vi "主程序-复材超声C扫缺陷分析评定软件.vi"() -> ()   [LabVIEW 2018]
doc: "使用该模板构建用户界面事件处理设计模式。将模板应用于对话框及其它用户界面。用户也可创建并执行VI可按照与用户界面事件相同方式处理的用户定义事件。"
uses:
  <vilib>/Utility/NIReport.llb/Report Type.ctl
  <vilib>/addons/_office/_exclsub.llb/font.ctl
  <vilib>/Utility/NIReport.llb/HTML Report Image Alignment.ctl
  <vilib>/Utility/NIReport.llb/Append Report Text (str wrap).vi
  <vilib>/Utility/NIReport.llb/Append Image to Report (path wrap).vi
  <vilib>/addons/_office/word.llb/Word Easy Table (str).vi
  <vilib>/Utility/NIReport.llb/NI_report.lvclass
  <vilib>/Utility/NIReport.llb/Word/NI_Word.lvclass
  <vilib>/addons/_office/NI_ReportGenerationToolkit.lvlib
  <vilib>/Utility/NIReport.llb/NI_ReportGenerationCore.lvlib
  <vilib>/vision/NI_Vision_Development_Module.lvlib
panel:
  out "框号字体大小-":i16
  out "是否需要预处理":u16
  out "弥散类缺陷灰度阈值":dbl caption="值"
  out "计入分层缺陷的面积阈值":i32
  out "报告模式":string
  in  "删除标注":bool caption="定量分析"
  out "分层类缺陷灰度阈值":dbl caption="值"
  out "反射图原始路径":path
  out "穿透图原始路径":path
  out "ROImask":T1(plugin-control)
  out "模式选择":u16(ring) items=["只读穿透图", "穿透图和反射图结合"]
  out "添加的路径":path
  out "连接的字符串 2":string
  out "临界面积百分比值":dbl
  out "临界Z值":i32
  out "标注后的图片路径":path
  out "全部检测结果合并":string[][](table)
  out "全部检测结果":string[][](table)
  out "部位信息":string[](array[string])=["", "34.500000", "32.500000", "1121", "34", "54.955926", "分层类", "不合格", ""]
  out "连接的字符串":string
  in  "完成标注":bool caption="定量分析"
  out "框数":dbl
  out "自定义字体":T2={"Desired Font (Application)"=enum."Application Font", "[User-specified Font]"={"Font Name"="", "Size"=12, "Strikeout?"=FALSE, "Italic?"=FALSE, "Underline?"=FALSE, "Outline?"=FALSE, "Shadow?"=FALSE, "Bold?"=FALSE, "Rotation Angle"=0.0}, "Horizontal Alignment"=0, "Vertical Alignment"=0} {"Horizontal Alignment" items=["Left", "Center", "Right"]; "Vertical Alignment" items=["Bottom", "Top", "Baseline"]}
  out "框组":T3(array[cluster])
  out "质量等级":string
  in  "stop":bool caption="停止"
  in  "导入图像":bool caption="导入图片"
  in  "开始标注":bool caption="定量分析"
  in  "查看评定结果":bool caption="辅助定性分析"
  in  "生成报告":bool caption="生成原始记录"
  in  "控件":enum32{"穿透图", "反射图"}(tab)
  out "穿透图":T1(plugin-control)
  out "反射图":T1(plugin-control)
  out "产品规格":cluster{"产品长度（周长）（mm）":dbl, "产品宽度（母线长）（mm）":dbl}
  out "图像分辨率":T4
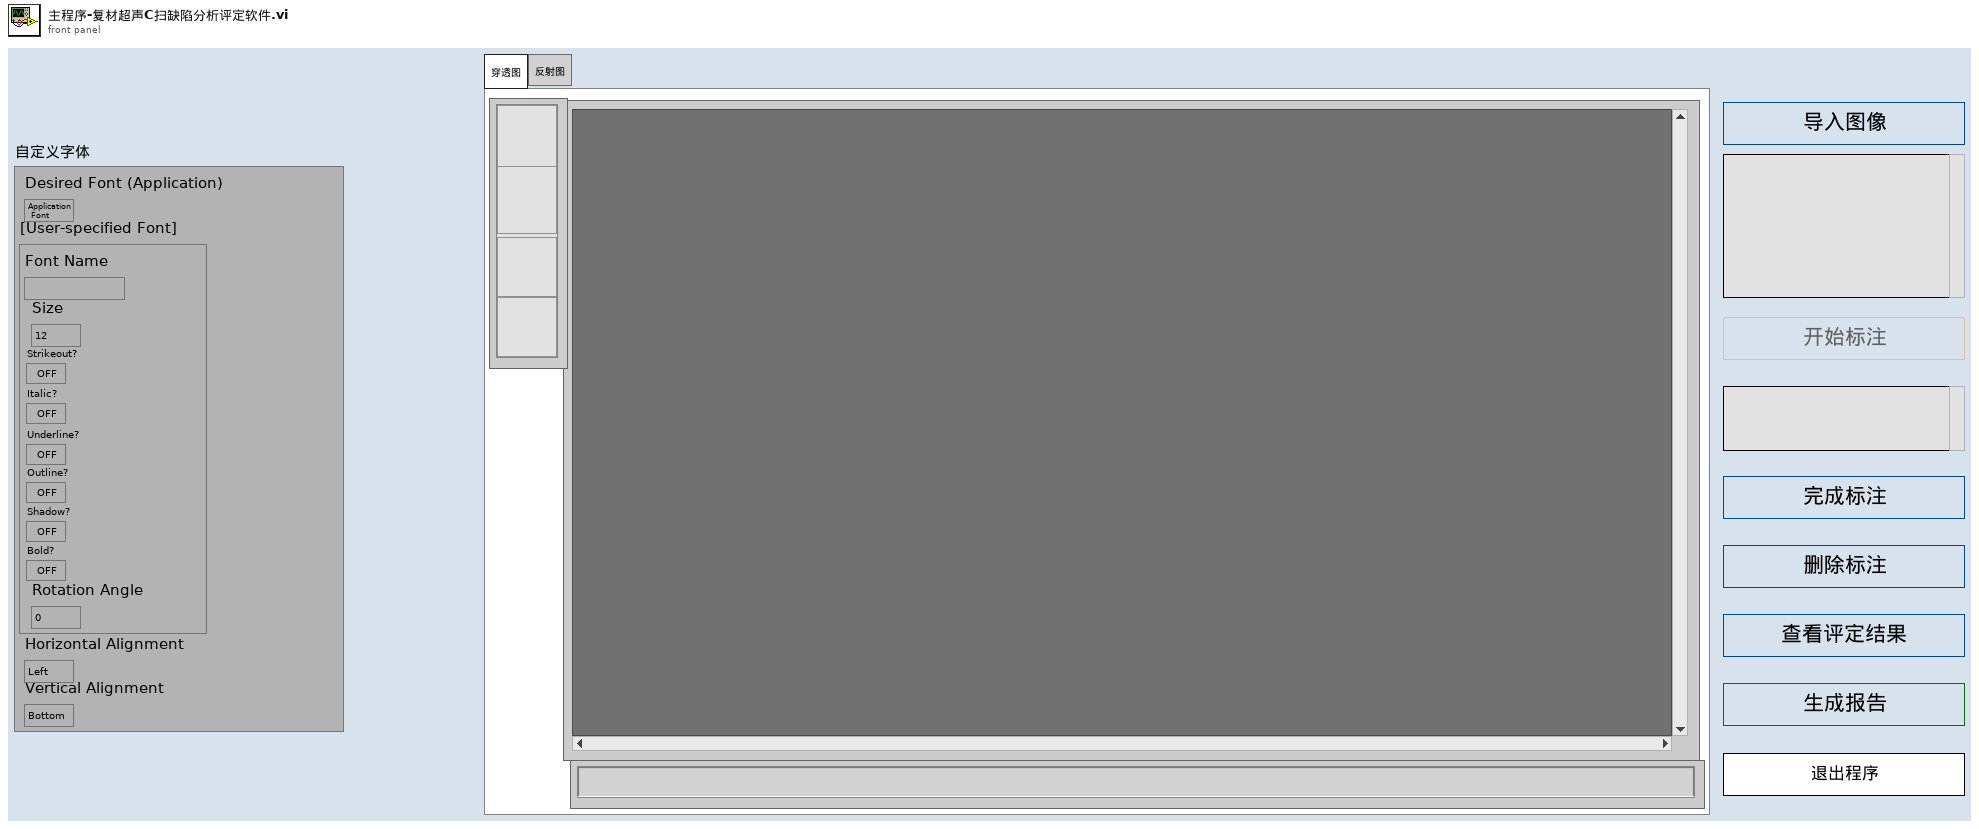
[diagram p1: front panel]
types:
  T1 = typedef "IMAQ Image.ctl" = refnum<image>
  T2 = cluster{"Desired Font (Application)":enum16{"User-specified Font", "Application Font", "System Font", "Dialog Font"}, "[User-specified Font]":cluster{"Font Name":string, "Size":i16, "Strikeout?":bool, "Italic?":bool, "Underline?":bool, "Outline?":bool, "Shadow?":bool, "Bold?":bool, "Rotation Angle":dbl}, "Horizontal Alignment":i16, "Vertical Alignment":i16}
  T3 = cluster{"Global Rectangle":i32[], "Contours":cluster{"Contour Type":u32, "ROI Type":u32, "Points":i32[]}[]}[]
  T4 = cluster{"图像X向分辨率（mm/像素）":dbl, "图像Y向分辨率（mm/像素）":dbl}
  T5 = enum8{"Enabled", "Disabled", "Disabled and Grayed Out"}
  T6 = cluster{"Global Rectangle":i32[], "Contours":cluster{"Contour Type":u32, "ROI Type":u32, "Points":i32[]}[]}
  T7 = cluster{"Zoom Tool":bool, "Selection Tool":bool, "Pan Tool":bool, "Point Tool":bool, "Line Tool":bool, "Rectangle Tool":bool, "Rotated Rectangle Tool":bool, "Polyline Tool":bool, "Polygon Tool":bool, "Freehand Tool":bool, "Closed Freehand Tool":bool, "Ellipse Tool":bool, "Annulus Tool":bool}
  T8 = enum16{"maximized", "minimized", "normal", "no change"}
  T9 = typedef "NI_ReportGenerationCore.lvlib/Report Type.ctl" = enum16{"HTML", "Word", "Excel"}
  T10 = typedef "NI_ReportGenerationCore.lvlib/HTML Report Image Alignment.ctl" = enum16{"(default)", "LEFT", "RIGHT", "TOP", "TEXTTOP", "MIDDLE", "ABSMIDDLE", "BASELINE", "BOTTOM", "ABSBOTTOM"}
  T11 = cluster{"position (Excel)":cluster{"row":i32, "column":i32}, "name (Excel)":string, "bookmark (Word)":string}
  T12 = cluster{"position (excel)":cluster{"row":i32, "column":i32}, "name (excel)":string, "bookmark (word)":string}
  T13 = typedef "NI_ReportGenerationToolkit.lvlib/font.ctl" = cluster{"font name":string, "font size":dbl, "bold":u16, "italic":u16, "underline":u16, "strike through":u16, "font color":u32}
  T14 = typedef "Image Type" = u32
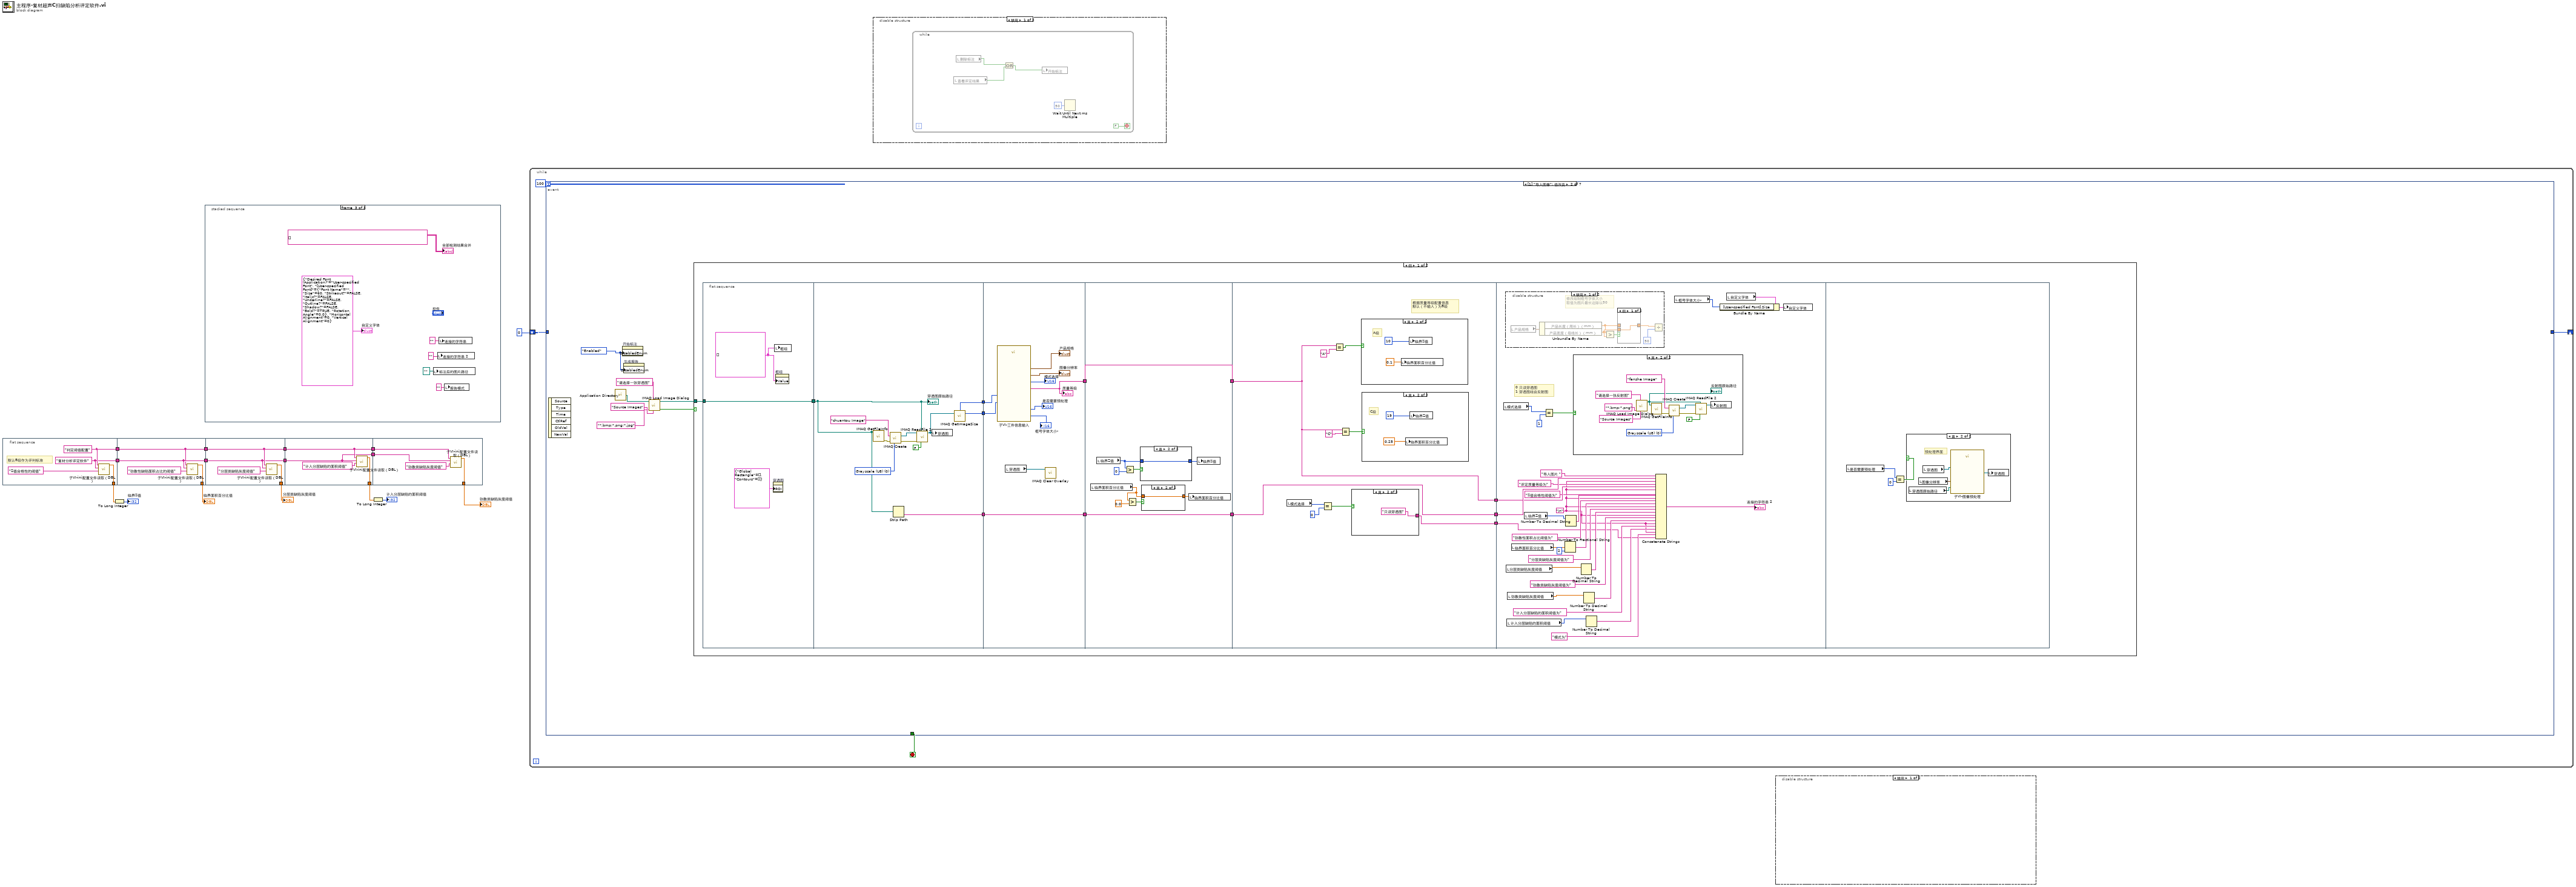
[diagram p0: block diagram]
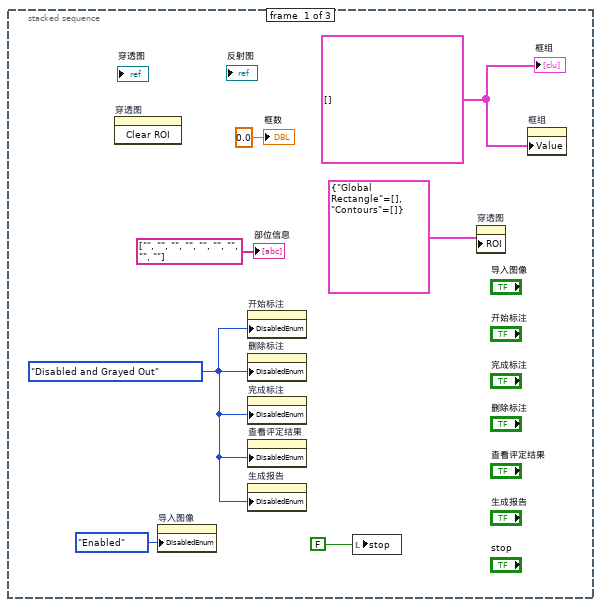
[diagram p3: hidden frame]
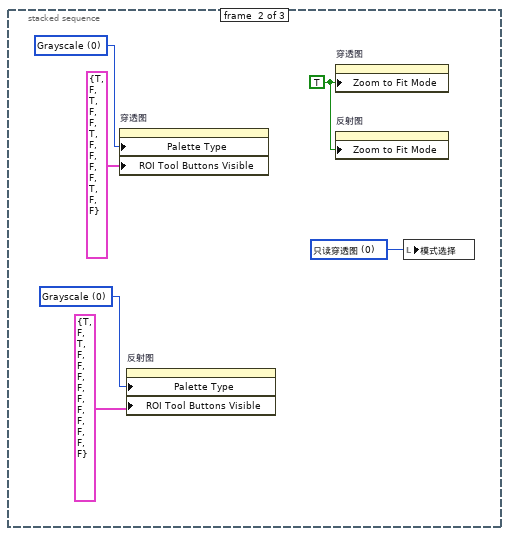
[diagram p4: hidden frame]
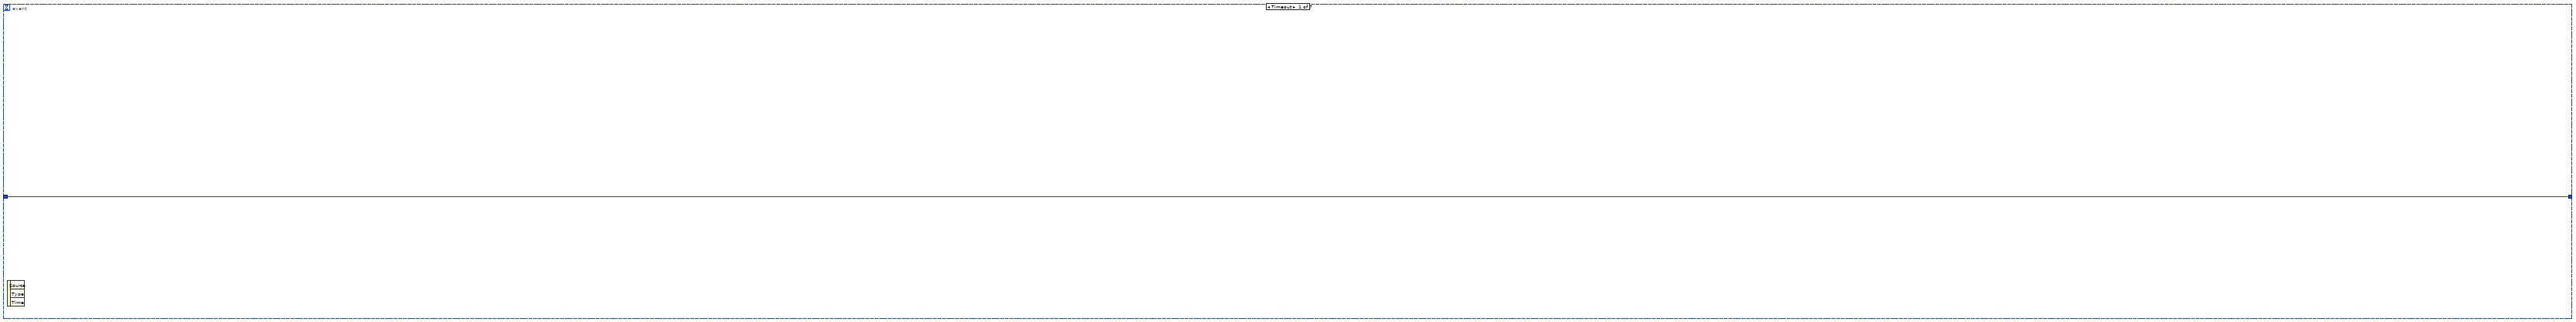
[diagram p6: hidden frame]
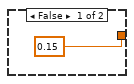
[diagram p7: hidden frame]
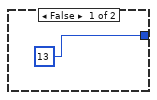
[diagram p8: hidden frame]
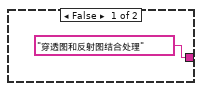
[diagram p9: hidden frame]
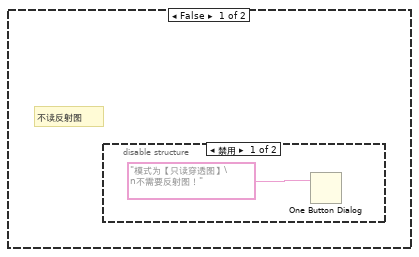
[diagram p14: hidden frame]
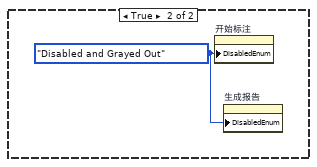
[diagram p17: hidden frame]
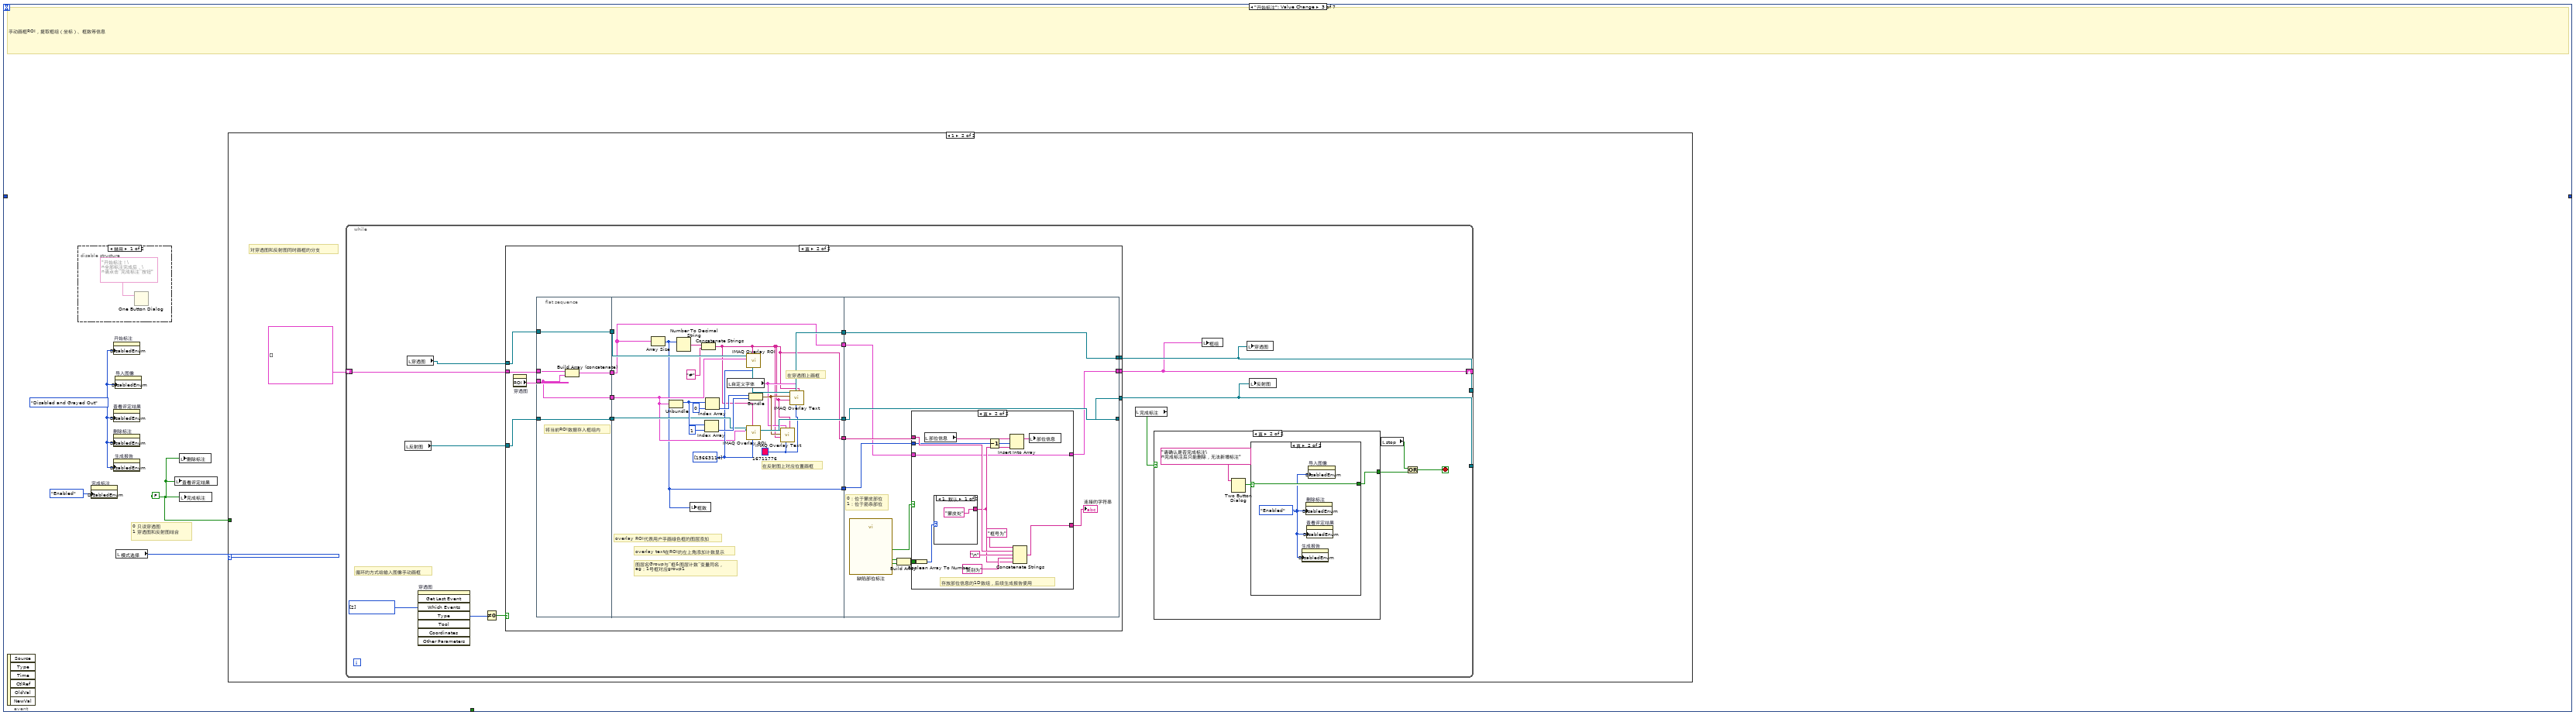
[diagram p18: hidden frame]
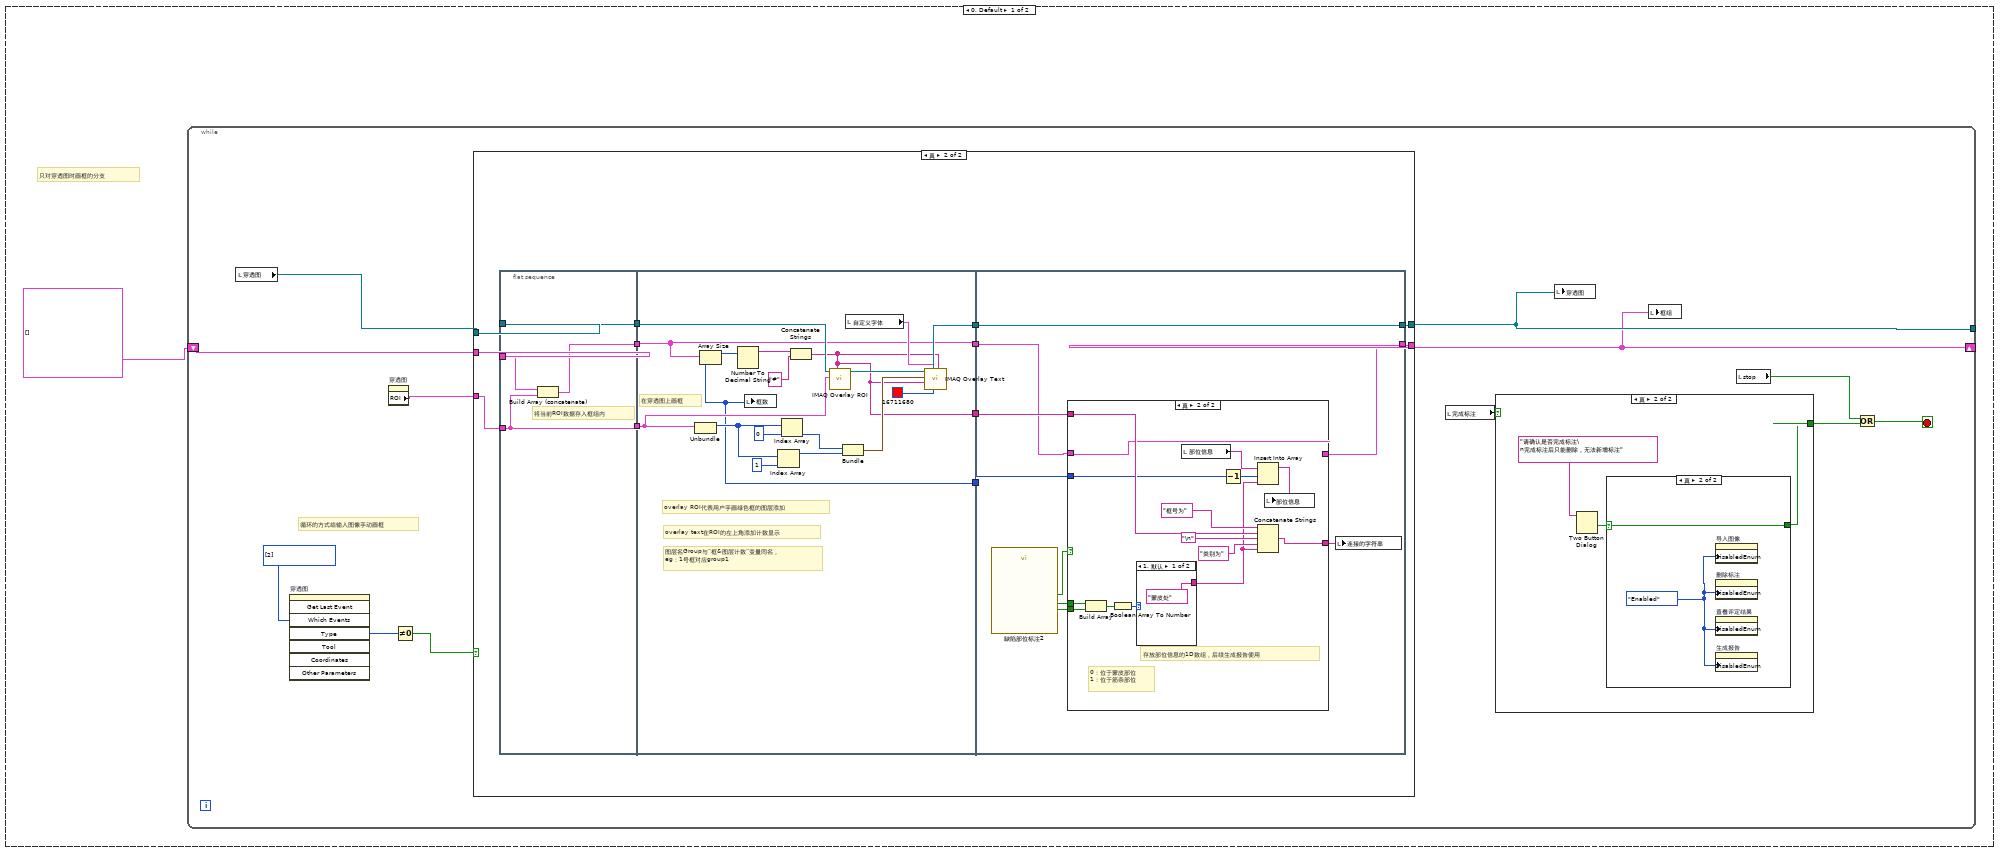
[diagram p20: hidden frame]
diagram:
  n1 = flat-sequence {
    tunnel: [w19] -> w15
    tunnel: [w18] -> w14
    tunnel: [w17] -> w9
    tunnel: w15 -> [w22]
    tunnel: w14 -> [w23]
    tunnel: [w23] -> w13
    tunnel: [w22] -> w12
    tunnel: [w21] -> w10
    tunnel: w13 -> [w25]
    tunnel: w12 -> [w26]
    tunnel: [w27] -> w11
    tunnel: [w26] -> w7
    tunnel: [w25] -> w6
    tunnel: w7 -> [w30]
    tunnel: w6 -> [w29]
    tunnel: [w31] -> w4
    tunnel: [w30] -> w3
    tunnel: [w29] -> w2
    tunnel: w3 -> [w35]
    tunnel: w2 -> [w34]
    tunnel: [w33] -> w1
    frame #0 {
      w18 = "复材分析评定软件" ("section")
      w19 = "判定阈值配置" ("文件名称")
      # "默认B级作为评判标准"
      n2 = call "子VI-ini配置文件读取（DBL）.vi"("key"="Z值合格性的阈值", "section"=w18, "文件名称"=w19) -> ("value"=w17:dbl)  [unwired: 8 in]
    }
    frame #1 {
      n3 = call "子VI-ini配置文件读取（DBL）.vi"("key"="弥散性缺陷面积占比的阈值", "section"=w23, "文件名称"=w22) -> ("value"=w21:dbl)  [unwired: 8 in]
    }
    frame #2 {
      n4 = call "子VI-ini配置文件读取（DBL）.vi"("key"="分层类缺陷灰度阈值", "section"=w25, "文件名称"=w26) -> ("value"=w27:dbl)  [unwired: 8 in]
    }
    frame #3 {
      n5 = call "子VI-ini配置文件读取（DBL）.vi"("key"="计入分层缺陷的面积阈值", "section"=w29, "文件名称"=w30) -> ("value"=w31:dbl)  [unwired: 8 in]
    }
    frame #4 {
      n6 = call "子VI-ini配置文件读取（DBL）.vi"("key"="弥散类缺陷灰度阈值", "section"=w34, "文件名称"=w35) -> ("value"=w33:dbl)  [unwired: 8 in]
    }
  }
  n7 = To Long Integer(number=w9) -> (32bit integer=→"临界Z值":i32)
  n8 = stacked-sequence {
    frame #0 {
      w41 = T3 [] ("框组")
      w38 = T5."Disabled and Grayed Out" ("禁用")
      n9 = invoke on="穿透图" class="ImageControl" method="Clear ROI"() -> ()  [unwired: 3 in, 3 out]
      n10 = property on="导入图像" class="Bool"("DisabledEnum"=T5."Enabled" ("禁用")) -> ()  [unwired: 2 in, 2 out]
      n11 = property on="开始标注" class="Bool"("DisabledEnum"=w38) -> ()  [unwired: 2 in, 2 out]
      n12 = property on="删除标注" class="Bool (严格)"("DisabledEnum"=w38) -> ()  [unwired: 2 in, 2 out]
      n13 = property on="完成标注" class="Bool (严格)"("DisabledEnum"=w38) -> ()  [unwired: 2 in, 2 out]
      n14 = property on="查看评定结果" class="Bool (严格)"("DisabledEnum"=w38) -> ()  [unwired: 2 in, 2 out]
      n15 = property on="生成报告" class="Bool"("DisabledEnum"=w38) -> ()  [unwired: 2 in, 2 out]
      n16 = local write "stop"(FALSE ("stop")) -> ()
      n17 = property on="穿透图" class="ImageControl"("ROI"=T6 {"Global Rectangle"=[], "Contours"=[]}) -> ()  [unwired: 2 in, 2 out]
      n18 = property on="框组" class="Arr (严格)"("Value"=w41) -> ()  [unwired: 2 in, 2 out]
      "部位信息" <- string[] ["", "", "", "", "", "", "", "", ""] ("部位信息")
      "框组" <- w41
      "框数" <- 0.0 ("框数")
    }
    frame #1 {
      w44 = u16 0 items=["只读穿透图", "穿透图和反射图结合"] ("模式选择")
      w46 = u32 0 items=["Grayscale", "Binary", "Gradient", "Rainbow", "Temperature", "User Defined", "Binary 16 Bit", "Gradient 16 Bit", "Rainbow 16 Bit", "Temperature 16 Bit", "User Defined 16 Bit"] ("Palette:Palette Type")
      w47 = TRUE ("Zoom to Fit Mode")
      w49 = u32 0 items=["Grayscale", "Binary", "Gradient", "Rainbow", "Temperature", "User Defined", "Binary 16 Bit", "Gradient 16 Bit", "Rainbow 16 Bit", "Temperature 16 Bit", "User Defined 16 Bit"] ("Palette:Palette Type")
      n19 = property on="穿透图" class="ImageControl"("Palette Type"=w49, "ROI Tool Buttons Visible"=T7 {"Zoom Tool"=TRUE, "Selection Tool"=FALSE, "Pan Tool"=TRUE, "Point Tool"=FALSE, "Line Tool"=FALSE, "Rectangle Tool"=TRUE, "Rotated Rectangle Tool"=FALSE, "Polyline Tool"=FALSE, "Polygon Tool"=FALSE, "Freehand Tool"=FALSE, "Closed Freehand Tool"=TRUE, "Ellipse Tool"=FALSE, "Annulus Tool"=FALSE} ("ROI Tool Buttons Visible:All Elements")) -> ()  [unwired: 2 in, 2 out]
      n20 = property on="反射图" class="ImageControl"("Palette Type"=w46, "ROI Tool Buttons Visible"=T7 {"Zoom Tool"=TRUE, "Selection Tool"=FALSE, "Pan Tool"=TRUE, "Point Tool"=FALSE, "Line Tool"=FALSE, "Rectangle Tool"=FALSE, "Rotated Rectangle Tool"=FALSE, "Polyline Tool"=FALSE, "Polygon Tool"=FALSE, "Freehand Tool"=FALSE, "Closed Freehand Tool"=FALSE, "Ellipse Tool"=FALSE, "Annulus Tool"=FALSE} ("ROI Tool Buttons Visible:All Elements")) -> ()  [unwired: 2 in, 2 out]
      n21 = property on="穿透图" class="ImageControl"("Zoom to Fit Mode"=w47) -> ()  [unwired: 2 in, 2 out]
      n22 = property on="反射图" class="ImageControl"("Zoom to Fit Mode"=w47) -> ()  [unwired: 2 in, 2 out]
      n23 = local write "模式选择"(w44) -> ()
    }
    frame #2 {
      n24 = local write "标注后的图片路径"(path "" ("标注后的图片路径")) -> ()
      n25 = local write "连接的字符串 2"("" ("连接的字符串 2")) -> ()
      n26 = local write "连接的字符串"("" ("连接的字符串")) -> ()
      n27 = local write "报告模式"("" ("报告模式")) -> ()
      "自定义字体" <- T2 {"Desired Font (Application)"=enum."User-specified Font", "[User-specified Font]"={"Font Name"="", "Size"=60, "Strikeout?"=FALSE, "Italic?"=FALSE, "Underline?"=FALSE, "Outline?"=FALSE, "Shadow?"=FALSE, "Bold?"=TRUE, "Rotation Angle"=0.0}, "Horizontal Alignment"=0, "Vertical Alignment"=0} ("Font, Size & Style")
      "全部检测结果合并" <- string[][] [] ("弥散类检测结果合并")
    }
  }
  n28 = To Long Integer(number=w4) -> (32bit integer=→"计入分层缺陷的面积阈值":i32)
  n29 = while {
    shift-right: [w56] -> _
    shift-left: 0 -> [w57]
    stop <- w59 stop-if-true
    n30 = event shown="[1] \"导入图像\": 值改变" {
      selector: _ -> [_ _ _ _ _ _ _]
      dyn-events: _ -> [_ _ _ _ _ _ _]
      timeout: 100 -> [_ _ _ _ _ _ _]
      tunnel: [_ _ _ _ _ _ w644] -> w59
      tunnel: w57 -> [w60 _ _ _ _ w441 _]
      tunnel: [w60 _ _ _ _ w441 0] -> w56
      event Timeout {
        n31 = event-data() -> ()  [unwired: 1 in, 3 out]
      }
      event "导入图像": Value Change {
        w62 = T5."Enabled" ("禁用")
        n32 = event-data() -> ()  [unwired: 1 in, 6 out]
        n33 = call <vilib>:"Application Directory.vi"() -> ("Application Directory"=w61:path)
        n34 = property on="开始标注" class="Bool"("DisabledEnum"=w62) -> ()  [unwired: 2 in, 2 out]
        n35 = property on="生成报告" class="Bool"("DisabledEnum"=w62) -> ()  [unwired: 2 in, 2 out]
        n36 = call "IMAQ Load Image Dialog"("Pattern Label"="Source Images", "Prompt"="请选择一张穿透图" ("prompt"), "Pattern"="*.bmp;*.png;*.jpg", "Start Path"=w61) -> ("Cancelled?"=w64:bool, "Path"=w63:path)  [unwired: 5 in, 1 out]
        n37 = case shown="假" w64 {
          tunnel: w63 -> [w77 _]
          frame False {
            n38 = flat-sequence {
              tunnel: w77 -> [w80]
              tunnel: [w80] -> w76
              tunnel: w76 -> [w84]
              tunnel: [w86] -> w75
              tunnel: [w85] -> w74
              tunnel: [w83] -> w73
              tunnel: [w100] -> w79
              tunnel: w75 -> [w99]
              tunnel: w74 -> [w98]
              tunnel: w73 -> [w97]
              tunnel: [w97] -> w72
              tunnel: w79 -> [w113]
              tunnel: [w113] -> w78
              tunnel: w72 -> [w112]
              tunnel: [w112] -> w71
              tunnel: w78 -> [w119]
              tunnel: w71 -> [w120]
              tunnel: [w120] -> w70
              tunnel: [w119] -> w69
              tunnel: [w118] -> w68
              tunnel: w70 -> [w151]
              tunnel: w69 -> [w149]
              tunnel: w68 -> [w137]
              frame #0 {
                w81 = T3 [] ("框组")
                n39 = property on="穿透图" class="ImageControl"("ROI"=T6 {"Global Rectangle"=[], "Contours"=[]}) -> ()  [unwired: 2 in, 2 out]
                n40 = local write "框组"(w81) -> ()
                n41 = property on="框组" class="Arr (严格)"("Value"=w81) -> ()  [unwired: 2 in, 2 out]
              }
              frame #1 {
                w88 = T14 0 items=["Grayscale (U8)", "Grayscale (I16)", "Grayscale (SGL)", "Complex (CSG)", "RGB (U32)", "HSL (U32)", "RGB (U64)", "Grayscale (U16)"] ("Image Type")
                n42 = call "IMAQ GetFileInfo"("File Path"=w84) -> ("error out"=w91:errorcluster)  [unwired: 4 in, 6 out]
                n43 = call "IMAQ Create"("Image Name"="chuantou Image", "Image Type"=w88, "error in (no error)"=w91) -> ("New Image"=w92:T1, "error out"=w93:errorcluster)  [unwired: 2 in]
                n44 = Strip Path(path=w84) -> (name=w83:string)  [unwired: 1 out]
                n45 = call "IMAQ ReadFile 2"("Use File Path Image Type"=FALSE, "File Path"=w84, "error in (no error)"=w93, "Image"=w92) -> ("Image Out"=w90:T1)  [unwired: 3 in, 4 out]
                n46 = local write "穿透图"(w90) -> ()
                n47 = call "IMAQ GetImageSize"("Image"=w90) -> ("Y Resolution"=w85:i32, "X Resolution"=w86:i32)  [unwired: 3 in, 1 out]
                "穿透图原始路径" <- w84
              }
              frame #2 {
                n48 = call "子VI-工件信息输入.vi"("Y Resolution"=w98, "X Resolution"=w99) -> ("质量等级"=w100:string, "模式选择"=→"模式选择":u16, "框号字体大小-"=→"框号字体大小-":i16, "产品规格"=→"产品规格":cluster{"产品长度（周长）（mm）":dbl, "产品宽度（母线长）（mm）":dbl}, "是否需要预处理"=→"是否需要预处理":u16, "图像分辨率"=→"图像分辨率":T4)  [unwired: 4 in]
                "质量等级" <- w100
                n49 = local read "穿透图"() -> (w96:T1)
                n50 = call "IMAQ Clear Overlay"("Image"=w96) -> ()  [unwired: 9 in, 2 out]
              }
              frame #3 {
                n51 = local read "临界面积百分比值"() -> (w104:dbl)
                n52 = local read "临界Z值"() -> (w105:i32)
                n53 = Greater?(x=w105, y=0) -> (0:w110:bool)
                n54 = Greater?(x=w104, y=0.0) -> (0:w108:bool)
                n55 = case shown="真" w110 {
                  tunnel: [13 ("临界Z值") w117] -> w107
                  tunnel: w105 -> [_ w117]
                  frame False {
                  }
                  frame True {
                  }
                }
                n56 = case shown="真" w108 {
                  tunnel: [0.15 ("临界面积百分比值") w115] -> w106
                  tunnel: w104 -> [_ w115]
                  frame False {
                  }
                  frame True {
                  }
                }
                n57 = local write "临界面积百分比值"(w106) -> ()
                n58 = local write "临界Z值"(w107) -> ()
              }
              frame #4 {
                # "根据质量等级配置信息\n默认（不输入）为B级"
                n59 = local read "模式选择"() -> (w122:u16)
                n60 = Equal?(x=w122, y=u16 0) -> (x = y?=w121:bool)
                n61 = Equal?(x=w119, y="A") -> (x = y?=w126:bool)
                n62 = Equal?(x=w119, y="C") -> (x = y?=w127:bool)
                n63 = case shown="真" w121 {
                  tunnel: ["穿透图和反射图结合处理" ("字符串") "只读穿透图" ("字符串")] -> w118
                  frame False {
                  }
                  frame True {
                  }
                }
                n64 = case shown="真" w126 {
                  frame False {
                  }
                  frame True {
                    # "A级"
                    n65 = local write "临界面积百分比值"(0.1 ("临界面积百分比值")) -> ()
                    n66 = local write "临界Z值"(10 ("临界Z值")) -> ()
                  }
                }
                n67 = case shown="真" w127 {
                  frame False {
                  }
                  frame True {
                    # "C级"
                    n68 = local write "临界面积百分比值"(0.25 ("临界面积百分比值")) -> ()
                    n69 = local write "临界Z值"(19 ("临界Z值")) -> ()
                  }
                }
              }
              frame #5 {
                w139 = "\n"
                # "0 只读穿透图\n1 穿透图结合反射图"
                n70 = local read "模式选择"() -> (w162:u16)
                n71 = disable-structure shown="禁用" {
                  frame Disabled {
                    # "修改绘制框号字体大小\n取值为图片最长边除以50"
                    n72 = local read "产品规格"() -> (w165:cluster{"产品长度（周长）（mm）":dbl, "产品宽度（母线长）（mm）":dbl})
                    n73 = Unbundle By Name(w165) -> ("产品长度（周长）（mm）"=w167:dbl, "产品宽度（母线长）（mm）"=w168:dbl)
                    n74 = Greater?(x=w167, y=w168) -> (0:w166:bool)
                    n75 = case shown="假" w166 {
                      tunnel: w167 -> [_ w171]
                      tunnel: w168 -> [w170 _]
                      tunnel: [w170 w171] -> w169
                      frame False {
                      }
                      frame True {
                      }
                    }
                    n76 = Divide(x=w169, y=i8 50) -> ()  [unwired: 1 out]
                  }
                  frame Enabled {
                  }
                }
                n77 = local read "分层类缺陷灰度阈值"() -> (w159:dbl)
                n78 = local read "计入分层缺陷的面积阈值"() -> (w142:i32)
                n79 = local read "弥散类缺陷灰度阈值"() -> (w145:dbl)
                n80 = local read "临界面积百分比值"() -> (w157:dbl)
                n81 = local read "临界Z值"() -> (w155:i32)
                n82 = Equal?(x=w162, y=u16 1) -> (x = y?=w161:bool)
                n83 = Number To Fractional String(number=w157, precision (6)=i16 2 ("精度(6)")) -> (F-format string=w158:string)  [unwired: 2 in]
                n84 = Number To Decimal String(number=w155) -> (decimal integer string=w156:string)  [unwired: 1 in]
                n85 = case shown="真" w161 {
                  frame False {
                    # "不读反射图"
                    n86 = disable-structure shown="禁用" {
                      frame Disabled {
                        n87 = One Button Dialog(message="模式为【只读穿透图】\n不需要反射图！" ("消息")) -> ()  [unwired: 1 in, 1 out]
                      }
                      frame Enabled {
                      }
                    }
                  }
                  frame True {
                    w175 = T14 0 items=["Grayscale (U8)", "Grayscale (I16)", "Grayscale (SGL)", "Complex (CSG)", "RGB (U32)", "HSL (U32)", "RGB (U64)", "Grayscale (U16)"] ("Image Type")
                    n88 = call "IMAQ Load Image Dialog"("Pattern Label"="Source Images", "Prompt"="请选择一张反射图" ("prompt"), "Pattern"="*.bmp;*.png") -> ("Path"=w174:path)  [unwired: 6 in, 2 out]
                    "反射图原始路径" <- w174
                    n89 = call "IMAQ GetFileInfo"("File Path"=w174) -> ("error out"=w178:errorcluster)  [unwired: 4 in, 6 out]
                    n90 = call "IMAQ Create"("Image Name"="fanshe Image", "Image Type"=w175, "error in (no error)"=w178) -> ("New Image"=w179:T1, "error out"=w180:errorcluster)  [unwired: 2 in]
                    n91 = call "IMAQ ReadFile 2"("Use File Path Image Type"=FALSE, "File Path"=w174, "error in (no error)"=w180, "Image"=w179) -> ("Image Out"=w173:T1)  [unwired: 3 in, 4 out]
                    n92 = local write "反射图"(w173) -> ()
                  }
                }
                n93 = Number To Decimal String(number=w159) -> (decimal integer string=w160:string)  [unwired: 1 in]
                n94 = Number To Decimal String(number=w145) -> (decimal integer string=w143:string)  [unwired: 1 in]
                n95 = Number To Decimal String(number=w142) -> (decimal integer string=w140:string)  [unwired: 1 in]
                n96 = Concatenate Strings("导入图片 " ("字符串"), w151, w139, "评定质量等级为" ("字符串"), w149, w139, "Z值合格性阈值为" ("字符串"), w156, w139, "弥散性面积占比阈值为" ("字符串"), w158, w139, "分层类缺陷灰度阈值为" ("字符串"), w160, w139, "弥散类缺陷灰度阈值为" ("字符串"), w143, w139, "计入分层缺陷的面积阈值为" ("字符串"), w140, w139, "模式为" ("字符串"), w137) -> (→"连接的字符串 2":string)
                n97 = local read "框号字体大小-"() -> (w134:i16)
                n98 = local read "自定义字体"() -> (w135:T2)
                n99 = Bundle By Name(cluster=w135, "[User-specified Font].Size"=w134) -> (w136:T2)
                n100 = local write "自定义字体"(w136) -> ()
              }
              frame #6 {
                n101 = local read "是否需要预处理"() -> (w185:u16)
                n102 = Equal?(x=w185, y=u16 0) -> (x = y?=w186:bool)
                n103 = case shown="真" w186 {
                  frame False {
                  }
                  frame True {
                    # "预处理界面"
                    n104 = local read "穿透图原始路径"() -> (w187:path)
                    n105 = local read "图像分辨率"() -> (w188:T4)
                    n106 = local read "穿透图"() -> (w190:T1)
                    n107 = call "子VI-图像预处理.vi"("图像分辨率"=w188, "穿透图"=w190, "穿透图原始路径"=w187) -> ("穿透图out"=w189:T1)  [unwired: 8 in]
                    n108 = local write "穿透图"(w189) -> ()
                  }
                }
              }
            }
          }
          frame True {
            w191 = T5."Disabled and Grayed Out" ("禁用")
            n109 = property on="开始标注" class="Bool"("DisabledEnum"=w191) -> ()  [unwired: 2 in, 2 out]
            n110 = property on="生成报告" class="Bool"("DisabledEnum"=w191) -> ()  [unwired: 2 in, 2 out]
          }
        }
      }
      event "开始标注": Value Change {
        w192 = T5."Disabled and Grayed Out" ("禁用")
        w194 = FALSE ("完成标注")
        # "0 只读穿透图\n1 穿透图和反射图结合"
        # "手动画框ROI，提取框组（坐标）、框数等信息"
        n111 = event-data() -> ()  [unwired: 1 in, 6 out]
        n112 = disable-structure shown="禁用" {
          frame Disabled {
            n113 = One Button Dialog(message="开始标注！\n全部标注完成后，\n请点击“完成标注”按钮" ("消息")) -> ()  [unwired: 1 in, 1 out]
          }
          frame Enabled {
          }
        }
        n114 = property on="完成标注" class="Bool (严格)"("DisabledEnum"=T5."Enabled" ("禁用")) -> ()  [unwired: 2 in, 2 out]
        n115 = property on="查看评定结果" class="Bool (严格)"("DisabledEnum"=w192) -> ()  [unwired: 2 in, 2 out]
        n116 = property on="删除标注" class="Bool (严格)"("DisabledEnum"=w192) -> ()  [unwired: 2 in, 2 out]
        n117 = property on="生成报告" class="Bool"("DisabledEnum"=w192) -> ()  [unwired: 2 in, 2 out]
        n118 = property on="开始标注" class="Bool"("DisabledEnum"=w192) -> ()  [unwired: 2 in, 2 out]
        n119 = property on="导入图像" class="Bool"("DisabledEnum"=w192) -> ()  [unwired: 2 in, 2 out]
        n120 = local read "模式选择"() -> (w195:u16)
        n121 = local write "查看评定结果"(w194) -> ()
        n122 = local write "删除标注"(w194) -> ()
        n123 = local write "完成标注"(w194) -> ()
        n124 = case shown="1" w195 {
          tunnel: w194 -> [_ _]
          frame 0, Default {
            # "只对穿透图时画框的分支"
            n125 = while {
              shift-right: [w199] -> _
              shift-left: T3 [] ("框组") -> [w209]
              tunnel: [w207] -> _
              stop <- w198 stop-if-true
              (unwired) "_" ("名称或相对路径")
              (unwired) ".docx" ("名称或相对路径")
              w205 = i32[] [2] items=["No Event"=0, "Click Event"=1, "Draw Event"=2, "Size Event"=4, "Scroll Event"=5, "Double Click Event"=8] ("Which Events")
              # "循环的方式给输入图像手动画框"
              n126 = local read "穿透图"() -> (w208:T1)
              n127 = invoke on="穿透图" class="ImageControl" method="Get Last Event"("Which Events"=w205) -> ("Type"=w201:i32)  [unwired: 7 in, 7 out]
              n128 = property on="穿透图" class="ImageControl"() -> ("ROI"=w203:T6)  [unwired: 2 in, 2 out]
              n129 = Not Equal To 0?(x=w201) -> (x != 0?=w200:bool)
              n130 = case shown="真" w200 {
                tunnel: w208 -> [w220 w232]
                tunnel: [w220 w231] -> w207
                tunnel: [w218 w229] -> w199
                tunnel: w209 -> [w218 w230]
                tunnel: w203 -> [_ w228]
                frame False {
                  n131 = Wait (ms)(milliseconds to wait=u32 50 ("毫秒倍数")) -> ()  [unwired: 1 out]
                  n132 = Wait (ms)(milliseconds to wait=u32 50) -> ()  [unwired: 1 out]
                }
                frame True {
                  n133 = flat-sequence {
                    tunnel: w232 -> [w233]
                    tunnel: [w233] -> w227
                    tunnel: w228 -> [w236]
                    tunnel: [w236] -> w226
                    tunnel: w230 -> [w235]
                    tunnel: [w234] -> w225
                    tunnel: w227 -> [w245]
                    tunnel: w226 -> [w244]
                    tunnel: w225 -> [w237]
                    tunnel: [w247] -> w224
                    tunnel: [w237] -> w223
                    tunnel: [w241] -> w222
                    tunnel: [w239] -> w221
                    tunnel: w224 -> [w262]
                    tunnel: w223 -> [w256]
                    tunnel: w222 -> [w259]
                    tunnel: w221 -> [w258]
                    tunnel: [w262] -> w231
                    tunnel: [w255] -> w229
                    frame #0 {
                      # "将当前ROI数据存入框组内"
                      n134 = Build Array (concatenate)(w235, w236) -> (w234:T3)
                    }
                    frame #1 {
                      # "在穿透图上画框"
                      # "图层名Group与“框&图层计数”变量同名，\neg：1号框对应group1"
                      # "overlay text在ROI的左上角添加计数显示"
                      # "overlay ROI代表用户手画绿色框的图层添加"
                      n135 = Unbundle(w244) -> ("Global Rectangle"=w252:i32[])  [unwired: 1 out]
                      n136 = Array Size(array=w237) -> (size(s)=w239:i32)
                      n137 = Number To Decimal String(number=w239) -> (decimal integer string=w240:string)  [unwired: 1 in]
                      n138 = local write "框数"(w239) -> ()
                      n139 = Index Array(array=w252, index=1 ("索引")) -> (element=w250:i32)
                      n140 = Index Array(array=w252, index=0 ("索引")) -> (element=w251:i32)
                      n141 = Concatenate Strings(w240, "#" ("字符串")) -> (w241:string)
                      n142 = call "IMAQ Overlay ROI"("Group"=w241, "ROI Descriptor"=w244, "Image"=w245) -> ("Image Out"=w253:T1)  [unwired: 7 in, 1 out]
                      n143 = Bundle(w251, w250) -> (w246:cluster{i32, i32})  [unwired: 1 in]
                      n144 = local read "自定义字体"() -> (w243:T2)
                      n145 = call "IMAQ Overlay Text"("Group"=w241, "Text Color (black)"=u32 16711680, "Font, Size & Style"=w243, "String"=w241, "Origin"=w246, "Image"=w253) -> ("Image Out"=w247:T1)  [unwired: 4 in, 1 out]
                    }
                    frame #2 {
                      n146 = call "缺陷部位标注2"() -> ("位于筋条处"=w261:bool, "位于蒙皮处"=w260:bool, "确定"=w257:bool)  [unwired: 16 in, 1 out]
                      n147 = case shown="真" w257 {
                        tunnel: w261 -> [_ w278]
                        tunnel: w260 -> [_ w277]
                        tunnel: w259 -> [_ w273]
                        tunnel: w258 -> [_ w270]
                        tunnel: w256 -> [w265 w267]
                        tunnel: [w264 w267] -> w255
                        tunnel: ["由于点击取消，该框不参与统计" w266] -> w254
                        frame False {
                          # "取消 不把该框信息写入框组"
                          n148 = Delete From Array(array=w265) -> (array with subset deleted=w264:T3)  [unwired: 2 in, 1 out]
                        }
                        frame True {
                          # "0：位于蒙皮部位\n1：位于筋条部位"
                          # "存放部位信息的1D数组，后续生成报告使用"
                          n149 = Build Array(w277, w278) -> (w279:bool[])
                          n150 = Boolean Array To Number(Boolean array=w279) -> (number=w280:u32)
                          n151 = case shown="1, 默认" w280 {
                            tunnel: ["蒙皮处" ("t") "筋条处" ("t")] -> w268
                            frame 1, Default {
                            }
                            frame 2 {
                            }
                          }
                          n152 = local read "部位信息"() -> (w272:string[])
                          n153 = Decrement(x=w270) -> (x-1=w269:i32)
                          n154 = Insert Into Array(array=w272, index=w269, new element=w268) -> (w271:string[])
                          n155 = Concatenate Strings("框号为" ("字符串"), w273, "\n", "类别为" ("字符串"), w268) -> (w266:string)
                          n156 = local write "部位信息"(w271) -> ()
                        }
                      }
                      n157 = local write "连接的字符串"(w254) -> ()
                    }
                  }
                }
              }
              n158 = local read "完成标注"() -> (w204:bool)
              n159 = case shown="真" w204 {
                tunnel: [FALSE ("T button?") w211] -> w202
                frame False {
                }
                frame True {
                  n160 = Two Button Dialog(message="请确认是否完成标注\n完成标注后只能删除，无法新增标注" ("消息")) -> (T button?=w212:bool)  [unwired: 2 in]
                  n161 = case shown="真" w212 {
                    selector: w212 -> [_ w216]
                    tunnel: [FALSE w216] -> w211
                    frame False {
                    }
                    frame True {
                      w215 = T5."Enabled" ("禁用")
                      n162 = property on="导入图像" class="Bool"("DisabledEnum"=w215) -> ()  [unwired: 2 in, 2 out]
                      n163 = property on="删除标注" class="Bool (严格)"("DisabledEnum"=w215) -> ()  [unwired: 2 in, 2 out]
                      n164 = property on="查看评定结果" class="Bool (严格)"("DisabledEnum"=w215) -> ()  [unwired: 2 in, 2 out]
                      n165 = property on="生成报告" class="Bool"("DisabledEnum"=w215) -> ()  [unwired: 2 in, 2 out]
                    }
                  }
                }
              }
              n166 = local write "穿透图"(w207) -> ()
              n167 = local write "框组"(w199) -> ()
              n168 = local read "stop"() -> (w206:bool)
              n169 = Or(x=w206, y=w202) -> (x .or. y?=w198:bool)
              n170 = call <vilib>:"Application Directory.vi"() -> ()  [unwired: 1 out]
            }
          }
          frame 1 {
            # "对穿透图和反射图同时画框的分支"
            n171 = while {
              shift-right: [w286] -> _
              shift-left: T3 [] ("框组") -> [w295]
              tunnel: [w293] -> _
              tunnel: [w292] -> _
              stop <- w285 stop-if-true
              (unwired) "_" ("名称或相对路径")
              (unwired) ".docx" ("名称或相对路径")
              w291 = i32[] [2] items=["No Event"=0, "Click Event"=1, "Draw Event"=2, "Size Event"=4, "Scroll Event"=5, "Double Click Event"=8] ("Which Events")
              # "循环的方式给输入图像手动画框"
              n172 = local read "反射图"() -> (w294:T1)
              n173 = local read "穿透图"() -> (w288:T1)
              n174 = invoke on="穿透图" class="ImageControl" method="Get Last Event"("Which Events"=w291) -> ("Type"=w290:i32)  [unwired: 7 in, 7 out]
              n175 = Not Equal To 0?(x=w290) -> (x != 0?=w296:bool)
              n176 = case shown="真" w296 {
                tunnel: w288 -> [w307 w323]
                tunnel: [w307 w308] -> w293
                tunnel: [w306 w318] -> w286
                tunnel: w295 -> [w306 w322]
                tunnel: w294 -> [w305 w321]
                tunnel: [w305 w320] -> w292
                frame False {
                  n177 = Wait (ms)(milliseconds to wait=u32 50 ("毫秒倍数")) -> ()  [unwired: 1 out]
                }
                frame True {
                  n178 = property on="穿透图" class="ImageControl"() -> ("ROI"=w319:T6)  [unwired: 2 in, 2 out]
                  n179 = flat-sequence {
                    tunnel: w323 -> [w326]
                    tunnel: [w326] -> w317
                    tunnel: w319 -> [w328]
                    tunnel: [w328] -> w316
                    tunnel: w322 -> [w327]
                    tunnel: w321 -> [w325]
                    tunnel: [w325] -> w315
                    tunnel: [w324] -> w314
                    tunnel: w317 -> [w337]
                    tunnel: w316 -> [w336]
                    tunnel: w315 -> [w342]
                    tunnel: w314 -> [w329]
                    tunnel: [w343] -> w313
                    tunnel: [w341] -> w312
                    tunnel: [w329] -> w311
                    tunnel: [w333] -> w310
                    tunnel: [w331] -> w309
                    tunnel: w313 -> [w352]
                    tunnel: w312 -> [w360]
                    tunnel: w311 -> [w354]
                    tunnel: w310 -> [w356]
                    tunnel: w309 -> [w355]
                    tunnel: [w360] -> w320
                    tunnel: [w353] -> w318
                    tunnel: [w352] -> w308
                    frame #0 {
                      # "将当前ROI数据存入框组内"
                      n180 = Build Array (concatenate)(w327, w328) -> (w324:T3)
                    }
                    frame #1 {
                      w339 = u32[] [15663114] ("Colors (Green)")
                      w335 = u32 16711776 ("Text Color (black)")
                      # "在反射图上对应位置画框"
                      # "在穿透图上画框"
                      # "图层名Group与“框&图层计数”变量同名，\neg：1号框对应group1"
                      # "overlay text在ROI的左上角添加计数显示"
                      # "overlay ROI代表用户手画绿色框的图层添加"
                      n181 = Array Size(array=w329) -> (size(s)=w331:i32)
                      n182 = Unbundle(w336) -> ("Global Rectangle"=w348:i32[])  [unwired: 1 out]
                      n183 = Number To Decimal String(number=w331) -> (decimal integer string=w332:string)  [unwired: 1 in]
                      n184 = local write "框数"(w331) -> ()
                      n185 = Concatenate Strings(w332, "#" ("字符串")) -> (w333:string)
                      n186 = Index Array(array=w348, index=1 ("索引")) -> (element=w346:i32)
                      n187 = Index Array(array=w348, index=0 ("索引")) -> (element=w347:i32)
                      n188 = local read "自定义字体"() -> (w334:T2)
                      n189 = call "IMAQ Overlay ROI"("Colors (Green)"=w339, "Group"=w333, "ROI Descriptor"=w336, "Image"=w337) -> ("Image Out"=w349:T1)  [unwired: 6 in, 1 out]
                      n190 = call "IMAQ Overlay ROI"("Colors (Green)"=w339, "Group"=w333, "ROI Descriptor"=w336, "Image"=w342) -> ("Image Out"=w340:T1)  [unwired: 6 in, 1 out]
                      n191 = Bundle(w347, w346) -> (w338:cluster{i32, i32})  [unwired: 1 in]
                      n192 = call "IMAQ Overlay Text"("Group"=w333, "Text Color (black)"=w335, "Font, Size & Style"=w334, "String"=w333, "Origin"=w338, "Image"=w340) -> ("Image Out"=w341:T1)  [unwired: 4 in, 1 out]
                      n193 = call "IMAQ Overlay Text"("Group"=w333, "Text Color (black)"=w335, "Font, Size & Style"=w334, "String"=w333, "Origin"=w338, "Image"=w349) -> ("Image Out"=w343:T1)  [unwired: 4 in, 1 out]
                    }
                    frame #2 {
                      # "0：位于蒙皮部位\n1：位于筋条部位"
                      n194 = call "缺陷部位标注"() -> ("位于筋条处"=w358:bool, "位于蒙皮处"=w357:bool, "确定"=w350:bool)  [unwired: 16 in, 1 out]
                      n195 = Build Array(w357, w358) -> (w359:bool[])
                      n196 = case shown="真" w350 {
                        tunnel: w359 -> [_ w375]
                        tunnel: w356 -> [_ w371]
                        tunnel: w355 -> [_ w368]
                        tunnel: w354 -> [w363 w365]
                        tunnel: [w362 w365] -> w353
                        tunnel: ["由于点击取消，该框不参与统计" w364] -> w351
                        frame False {
                          # "取消 不把该框信息写入框组"
                          n197 = Delete From Array(array=w363) -> (array with subset deleted=w362:T3)  [unwired: 2 in, 1 out]
                        }
                        frame True {
                          # "存放部位信息的1D数组，后续生成报告使用"
                          n198 = Boolean Array To Number(Boolean array=w375) -> (number=w376:u32)
                          n199 = local read "部位信息"() -> (w370:string[])
                          n200 = case shown="1, 默认" w376 {
                            tunnel: ["蒙皮处" ("t") "筋条处" ("t")] -> w366
                            frame 1, Default {
                            }
                            frame 2 {
                            }
                          }
                          n201 = Decrement(x=w368) -> (x-1=w367:i32)
                          n202 = Insert Into Array(array=w370, index=w367, new element=w366) -> (w369:string[])
                          n203 = Concatenate Strings("框号为" ("字符串"), w371, "\n", "类别为" ("字符串"), w366) -> (w364:string)
                          n204 = local write "部位信息"(w369) -> ()
                        }
                      }
                      "连接的字符串" <- w351
                    }
                  }
                }
              }
              n205 = local read "完成标注"() -> (w284:bool)
              n206 = case shown="真" w284 {
                tunnel: [FALSE ("T button?") w298] -> w287
                frame False {
                }
                frame True {
                  n207 = Two Button Dialog(message="请确认是否完成标注\n完成标注后只能删除，无法新增标注" ("消息")) -> (T button?=w299:bool)  [unwired: 2 in]
                  n208 = case shown="真" w299 {
                    selector: w299 -> [_ w303]
                    tunnel: [FALSE w303] -> w298
                    frame False {
                    }
                    frame True {
                      w302 = T5."Enabled" ("禁用")
                      n209 = property on="生成报告" class="Bool"("DisabledEnum"=w302) -> ()  [unwired: 2 in, 2 out]
                      n210 = property on="删除标注" class="Bool (严格)"("DisabledEnum"=w302) -> ()  [unwired: 2 in, 2 out]
                      n211 = property on="查看评定结果" class="Bool (严格)"("DisabledEnum"=w302) -> ()  [unwired: 2 in, 2 out]
                      n212 = property on="导入图像" class="Bool"("DisabledEnum"=w302) -> ()  [unwired: 2 in, 2 out]
                    }
                  }
                }
              }
              n213 = local write "框组"(w286) -> ()
              n214 = local write "穿透图"(w293) -> ()
              n215 = local write "反射图"(w292) -> ()
              n216 = local read "stop"() -> (w289:bool)
              n217 = Or(x=w289, y=w287) -> (x .or. y?=w285:bool)
              n218 = call <vilib>:"Application Directory.vi"() -> ()  [unwired: 1 out]
            }
          }
        }
      }
      event "删除标注": Value Change {
        w380 = T5."Disabled and Grayed Out" ("禁用")
        n219 = event-data() -> ()  [unwired: 1 in, 6 out]
        n220 = call "用户输入2"() -> ("框号"=w381:dbl, "确定"=w382:bool)  [unwired: 17 in, 1 out]
        n221 = property on="生成报告" class="Bool"("DisabledEnum"=T5."Enabled" ("禁用")) -> ()  [unwired: 2 in, 2 out]
        n222 = property on="完成标注" class="Bool (严格)"("DisabledEnum"=w380) -> ()  [unwired: 2 in, 2 out]
        n223 = property on="开始标注" class="Bool"("DisabledEnum"=w380) -> ()  [unwired: 2 in, 2 out]
        n224 = case shown="真" w382 {
          tunnel: w381 -> [_ w383]
          frame False {
            # "用户取消操作"
          }
          frame True {
            n225 = stacked-sequence {
              tunnel: w383 -> [_ w390 _]
              frame #0 {
                # "1. 删除所有框"
                n226 = local read "穿透图"() -> (w384:T1)
                n227 = call "IMAQ Clear Overlay"("Image"=w384) -> ()  [unwired: 9 in, 2 out]
              }
              frame #1 {
                # "2. 删除框组中指定元素"
                n228 = local read "部位信息"() -> (w387:string[])
                n229 = local read "框组"() -> (w389:T3)
                n230 = Decrement(x=w390) -> (x-1=w386:dbl)
                n231 = Delete From Array(array=w387, index=w386) -> (array with subset deleted=w385:string[])  [unwired: 1 in, 1 out]
                n232 = Delete From Array(array=w389, index=w386) -> (array with subset deleted=w388:T3)  [unwired: 1 in, 1 out]
                n233 = local write "框组"(w388) -> ()
                n234 = local write "部位信息"(w385) -> ()
              }
              frame #2 {
                # "3. 重画所有框"
                n235 = while {
                  i -> [w403]
                  stop <- w394 stop-if-true
                  n236 = local read "框组"() -> (w398:T3)
                  n237 = local read "穿透图"() -> (w402:T1)
                  n238 = Array Size(array=w398) -> (size(s)=w399:i32)
                  n239 = Index Array(array=w398, index=w403) -> (element=w393:T6)
                  n240 = Increment(x=w403) -> (x+1=w410:i32)
                  n241 = local write "框数"(w399) -> ()
                  n242 = Greater Or Equal?(x=w410, y=w399) -> (x >= y?=w394:bool)
                  n243 = call "IMAQ Overlay ROI"("ROI Descriptor"=w393, "Image"=w402) -> ("Image Out"=w408:T1)  [unwired: 8 in, 1 out]
                  n244 = Unbundle(w393) -> ("Global Rectangle"=w400:i32[])  [unwired: 1 out]
                  n245 = Number To Decimal String(number=w410) -> (decimal integer string=w395:string)  [unwired: 1 in]
                  n246 = Index Array(array=w400, index=0 ("索引")) -> (element=w405:i32)
                  n247 = Index Array(array=w400, index=1 ("索引")) -> (element=w406:i32)
                  n248 = local read "自定义字体"() -> (w392:T2)
                  n249 = Concatenate Strings(w395, "#" ("字符串")) -> (w391:string)
                  n250 = Bundle(w405, w406) -> (w396:cluster{i32, i32})  [unwired: 1 in]
                  n251 = call "IMAQ Overlay Text"("Text Color (black)"=u32 16711680, "Font, Size & Style"=w392, "String"=w391, "Origin"=w396, "Image"=w408) -> ("Image Out"=w401:T1)  [unwired: 5 in, 1 out]
                  n252 = local write "穿透图"(w401) -> ()
                }
              }
            }
          }
        }
      }
      event "查看评定结果": Value Change {
        w414 = T5."Disabled and Grayed Out" ("禁用")
        # "只读穿透图的图像处理方法"
        # "查看指定框的详细信息，包括灰度和面积阈值分割后的结果，提取到的长宽面积等信息"
        n253 = event-data() -> ()  [unwired: 1 in, 6 out]
        n254 = property on="完成标注" class="Bool (严格)"("DisabledEnum"=w414) -> ()  [unwired: 2 in, 2 out]
        n255 = property on="开始标注" class="Bool"("DisabledEnum"=w414) -> ()  [unwired: 2 in, 2 out]
        n256 = local read "计入分层缺陷的面积阈值"() -> (w412:i32)
        n257 = local read "弥散类缺陷灰度阈值"() -> (w413:dbl)
        n258 = local read "分层类缺陷灰度阈值"() -> (w415:dbl)
        n259 = local read "临界面积百分比值"() -> (w417:dbl)
        n260 = local read "穿透图原始路径"() -> (w420:path)
        n261 = local read "临界Z值"() -> (w418:i32)
        n262 = local read "部位信息"() -> (w422:string[])
        n263 = local read "产品规格"() -> (w421:cluster{"产品长度（周长）（mm）":dbl, "产品宽度（母线长）（mm）":dbl})
        n264 = local read "框组"() -> (w419:T3)
        n265 = call "子VI-查看某框-读穿透图模式.vi"("输入框号（默认值0为整张图）"=0.0 ("框号"), "框组"=w419, "临界Z值"=w418, "弥散类缺陷灰度阈值"=w413, "临界面积百分比值"=w417, "分层缺陷的面积阈值"=w412, "预先配置的灰度阈值"=w415, "穿透图原始路径"=w420, "部位信息"=w422, "产品规格"=w421) -> ("全部检测结果"=→"全部检测结果":string[][])  [unwired: 17 in]
      }
      event "生成报告": Value Change {
        w427 = T5."Disabled and Grayed Out" ("禁用")
        # "相当于“查看标注”一栏中的操作做循环，遍历所有框，\n将输出结果叠加为数组，作为最终结果输出并导入word"
        n266 = event-data() -> ()  [unwired: 1 in, 6 out]
        n267 = call "报告模式选择"() -> ("深度学习方法"=w426:bool, "自动检测结果"=w429:bool, "手动框选结果"=w430:bool, "确定"=w428:bool)  [unwired: 15 in, 1 out]
        n268 = local read "计入分层缺陷的面积阈值"() -> (w423:i32)
        n269 = local read "分层类缺陷灰度阈值"() -> (w433:dbl)
        n270 = Build Array(w430, w429, w426) -> (w432:bool[])
        n271 = local read "临界面积百分比值"() -> (w434:dbl)
        n272 = local read "弥散类缺陷灰度阈值"() -> (w424:dbl)
        n273 = local read "穿透图原始路径"() -> (w437:path)
        n274 = Boolean Array To Number(Boolean array=w432) -> (number=w431:u32)
        n275 = local read "模式选择"() -> (w440:u16)
        n276 = local read "产品规格"() -> (w438:cluster{"产品长度（周长）（mm）":dbl, "产品宽度（母线长）（mm）":dbl})
        n277 = local read "部位信息"() -> (w439:string[])
        n278 = local read "框组"() -> (w436:T3)
        n279 = property on="删除标注" class="Bool (严格)"("DisabledEnum"=w427) -> ()  [unwired: 2 in, 2 out]
        n280 = property on="完成标注" class="Bool (严格)"("DisabledEnum"=w427) -> ()  [unwired: 2 in, 2 out]
        n281 = property on="开始标注" class="Bool"("DisabledEnum"=w427) -> ()  [unwired: 2 in, 2 out]
        n282 = local read "临界Z值"() -> (w435:i32)
        n283 = case shown="真" w428 {
          tunnel: w440 -> [_ w455]
          tunnel: w439 -> [_ w454]
          tunnel: w438 -> [_ w453]
          tunnel: w437 -> [_ w452]
          tunnel: w436 -> [_ w451]
          tunnel: w435 -> [_ w450]
          tunnel: w434 -> [_ w449]
          tunnel: string[][] [] ("分层类检测结果合并 2") -> [_ w448]
          tunnel: w433 -> [_ w447]
          tunnel: w431 -> [_ w446]
          tunnel: w424 -> [_ w443]
          tunnel: w423 -> [_ w442]
          frame False {
          }
          frame True {
            n284 = case shown="0, 默认" w446 {
              tunnel: [w465 w491 w521 w535] -> w456
              tunnel: w455 -> [_ _ _ _]
              tunnel: w454 -> [w468 w499 w528 _]
              tunnel: w453 -> [w467 w498 w527 w540]
              tunnel: w452 -> [w469 w497 w526 w539]
              tunnel: w451 -> [w470 w496 w525 _]
              tunnel: w450 -> [w472 w493 w524 w538]
              tunnel: w449 -> [w473 w494 w523 w537]
              tunnel: w448 -> [w474 w492 w520 w536]
              tunnel: w447 -> [w471 w495 w522 w532]
              tunnel: w443 -> [w463 w490 w519 w531]
              tunnel: w442 -> [w462 w489 w518 w530]
              frame 0, Default {
                # "只读穿透图的图像处理方法"
                # "默认手动框选结果"
                n285 = local read "框数"() -> (w466:dbl)
                n286 = for {
                  N: w466 -> [_]
                  shift-right: [w488] -> w465
                  shift-left: w474 -> [w487]
                  tunnel: w468 -> [w484]
                  tunnel: w467 -> [w483]
                  tunnel: w469 -> [w482]
                  tunnel: w470 -> [w481]
                  tunnel: w473 -> [w480]
                  tunnel: w471 -> [w479]
                  tunnel: w472 -> [w478]
                  tunnel: w463 -> [w476]
                  tunnel: w462 -> [w475]
                  i -> [w486]
                  n287 = Increment(x=w486) -> (x+1=w485:i32)
                  n288 = call "子VI-查看某框-不显示界面-只读穿透图模式.vi"("框号"=w485, "框组"=w481, "分层缺陷的面积阈值"=w475, "临界Z值"=w478, "弥散类缺陷灰度阈值"=w476, "临界面积百分比值"=w480, "预先配置的灰度阈值"=w479, "穿透图原始路径"=w482, "部位信息"=w484, "产品规格"=w483) -> ("全部检测结果"=w477:string[][])  [unwired: 17 in]
                  n289 = Build Array (concatenate)(w487, w477) -> (w488:string[][])
                }
                "报告模式" <- "手动框选"
              }
              frame 1 {
                # "只读穿透图的图像处理方法"
                n290 = local read "框数"() -> (w500:dbl)
                n291 = local write "报告模式"("手动框选") -> ()
                n292 = for {
                  N: w500 -> [_]
                  shift-right: [w515] -> w491
                  shift-left: w492 -> [w514]
                  tunnel: w499 -> [w511]
                  tunnel: w498 -> [w510]
                  tunnel: w497 -> [w509]
                  tunnel: w496 -> [w508]
                  tunnel: w495 -> [w507]
                  tunnel: w494 -> [w506]
                  tunnel: w493 -> [w505]
                  tunnel: w490 -> [w503]
                  tunnel: w489 -> [w502]
                  i -> [w513]
                  n293 = Increment(x=w513) -> (x+1=w512:i32)
                  n294 = call "子VI-查看某框-不显示界面-只读穿透图模式.vi"("框号"=w512, "框组"=w508, "分层缺陷的面积阈值"=w502, "临界Z值"=w505, "弥散类缺陷灰度阈值"=w503, "临界面积百分比值"=w506, "预先配置的灰度阈值"=w507, "穿透图原始路径"=w509, "部位信息"=w511, "产品规格"=w510) -> ("全部检测结果"=w504:string[][])  [unwired: 17 in]
                  n295 = Build Array (concatenate)(w514, w504) -> (w515:string[][])
                }
              }
              frame 2 {
                # "只读穿透图的图像处理方法"
                n296 = local write "报告模式"("自动检测") -> ()
                n297 = call "子VI-查看某框-不显示界面-只读穿透图模式.vi"("框号"=0.0, "框组"=w525, "分层缺陷的面积阈值"=w518, "临界Z值"=w524, "弥散类缺陷灰度阈值"=w519, "临界面积百分比值"=w523, "预先配置的灰度阈值"=w522, "穿透图原始路径"=w526, "部位信息"=w528, "产品规格"=w527) -> ("全部检测结果"=w516:string[][])  [unwired: 17 in]
                n298 = Build Array (concatenate)(w520, w516) -> (w521:string[][])
              }
              frame 4 {
                # "深度学习方法自动检测demo"
                n299 = local write "报告模式"("深度学习自动检测" ("报告模式")) -> ()
                n300 = call "子VI-深度学习自动检测.vi"("临界Z值"=w538, "弥散类缺陷灰度阈值"=w531, "临界面积百分比值"=w537, "分层缺陷的面积阈值"=w530, "产品规格"=w540, "穿透图原始路径"=w539, "输入的灰度阈值"=w532) -> ("全部检测结果"=w533:string[][])  [unwired: 8 in]
                n301 = Build Array (concatenate)(w533, w536) -> (w535:string[][])
              }
            }
            n302 = local write "全部检测结果合并"(w456) -> ()
            n303 = flat-sequence {
              tunnel: w456 -> [w541]
              tunnel: [w541] -> w461
              tunnel: w461 -> [w582]
              tunnel: [w582] -> w460
              tunnel: w460 -> [w588]
              tunnel: [w588] -> w459
              tunnel: [w584] -> w445
              tunnel: [w583] -> w444
              tunnel: [w615] -> w458
              tunnel: [w614] -> w457
              tunnel: w459 -> [w608]
              tunnel: w445 -> [w605]
              tunnel: w444 -> [w604]
              tunnel: w457 -> [w634]
              tunnel: w458 -> [w635]
              frame #0 {
                n304 = while {
                  tunnel: [w559] -> _
                  i -> [w561]
                  stop <- w559 stop-if-true
                  w566 = 1 items=["White", "Black", "Inverted", "Black on White", "White on Black"] ("Color")
                  w568 = u16 2 items=["Frame", "Paint", "Invert Frame", "Invert Paint"] ("Draw Mode")
                  w563 = u16 1 items=["Line", "Rectangle", "Oval"] ("Shape to draw")
                  # "生成绘制了ROI的图像\n可以用于后续的图片导出保存"
                  n305 = local read "框组"() -> (w560:T3)
                  n306 = local read "ROImask"() -> (w556:T1)
                  n307 = local read "穿透图"() -> (w557:T1)
                  n308 = Array Size(array=w560) -> (size(s)=w569:i32)
                  n309 = Index Array(array=w560, index=w561) -> (element=w554:T6)
                  n310 = Unbundle By Name(w554) -> ("Global Rectangle"=w549:i32[])
                  n311 = Increment(x=w561) -> (x+1=w570:i32)
                  n312 = Greater Or Equal?(x=w570, y=w569) -> (x >= y?=w559:bool)
                  n313 = Index Array(array=w549, index=2 ("索引")) -> (element=w548:i32)
                  n314 = Index Array(array=w549, index=0 ("索引")) -> (element=w545:i32)
                  n315 = Index Array(array=w549, index=3 ("索引")) -> (element=w547:i32)
                  n316 = Index Array(array=w549, index=1 ("索引")) -> (element=w544:i32)
                  n317 = Number To Decimal String(number=w570) -> (decimal integer string=w564:string)  [unwired: 1 in]
                  n318 = Build Array(w545, w544, w548, w547) -> (w546:i32[])
                  n319 = call "IMAQ Draw"("Draw Mode"=w568, "Shape to draw"=w563, "Coordinates"=w546, "Image Src"=w557) -> ("Image Dst Out"=w567:T1)  [unwired: 6 in, 1 out]
                  n320 = Concatenate Strings(w564, "#" ("字符串")) -> (w562:string)
                  n321 = local read "自定义字体"() -> (w558:T2)
                  n322 = Build Array(w545, w544) -> (w543:i32[])
                  n323 = call "IMAQ Draw Text"("String"=w562, "Insertion Point"=w543, "Color"=w566, "Font, Size & Style"=w558, "Image Dst"=w556, "Image Src"=w567) -> ("error out"=w542:errorcluster, "Image Dst Out"=w555:T1)  [unwired: 2 in, 2 out]
                  "ROImask" <- w555
                  n324 = case shown="错误" w542 {
                    frame No Error {
                    }
                    frame Error {
                      n325 = One Button Dialog(message="失败！无法保存图片到报告" ("消息")) -> ()  [unwired: 1 in, 1 out]
                    }
                  }
                  n326 = local write "ROImask"(w555) -> ()
                }
              }
              frame #1 {
                n327 = local read "穿透图原始路径"() -> (w581:path)
                n328 = local read "ROImask"() -> (w573:T1)
                n329 = Path To String(path=w581) -> (string=w578:string)
                n330 = String Length(string=w578) -> (length=w579:i32)
                n331 = Subtract(x=w579, y=4) -> (x-y=w580:i32)
                n332 = Replace Substring(3:w580, 4:"_标注后.png" ("字符串"), 5:w578) -> (1:w577:string)  [unwired: 1 in, 1 out]
                n333 = String To Path(string=w577) -> (path=w572:path)
                "标注后的图片路径" <- w572
                n334 = call-poly "IMAQ Write File 2"("Image Quality"=u32 1000, "File Path"=w572, "Image"=w573) -> ()  [unwired: 7 in, 2 out]
              }
              frame #2 {
                # "最终检测结果全部合并 导入word中"
                n335 = call <vilib>:"Application Directory.vi"() -> ("Application Directory"=w587:path)
                n336 = Build Path(base path=w587, name or relative path="report-template.docx") -> (appended path=w585:path)
                n337 = call <vilib>:"Create Report.vi"("window state (normal)"=T8."maximized", "report type"=Report_Type."Word", "template (empty)"=w585) -> ("report out"=w584:refnum<class "NI_report.lvclass">, "error out"=w583:errorcluster)  [unwired: 11 in]
              }
              frame #3 {
                n338 = local read "报告模式"() -> (w606:string)
                n339 = local read "质量等级"() -> (w602:string)
                n340 = local read "标注后的图片路径"() -> (w595:path)
                n341 = Get Date/Time String(date format (0)=enum16{"short", "long", "abbreviated"}."long" ("日期格式(0)")) -> (date string=w612:string, time string=w613:string)  [unwired: 2 in]
                n342 = call-poly <vilib>:"Append Report Text.vi"("report in"=w605, "MS Office parameters"=T12 {"position (excel)"={"row"=0, "column"=0}, "name (excel)"="", "bookmark (word)"="mode"}, "text"=w606, "error in (no error)"=w604) -> ("report out"=w601:refnum<class "NI_report.lvclass">, "error out"=w600:errorcluster)  [unwired: 8 in, 2 out]
                n343 = Concatenate Strings(w612, w613) -> (w611:string)
                n344 = call-poly <vilib>:"Append Report Text.vi"("report in"=w601, "MS Office parameters"=T12 {"position (excel)"={"row"=0, "column"=0}, "name (excel)"="", "bookmark (word)"="class"}, "text"=w602, "error in (no error)"=w600) -> ("report out"=w598:refnum<class "NI_report.lvclass">, "error out"=w599:errorcluster)  [unwired: 8 in, 2 out]
                n345 = call-poly <vilib>:"Append Report Text.vi"("report in"=w598, "MS Office parameters"=T12 {"position (excel)"={"row"=0, "column"=0}, "name (excel)"="", "bookmark (word)"="time"}, "text"=w611, "error in (no error)"=w599) -> ("report out"=w593:refnum<class "NI_report.lvclass">, "error out"=w592:errorcluster)  [unwired: 8 in, 2 out]
                n346 = call-poly <vilib>:"Append Image to Report.vi"("report in"=w593, "alignment (default)"=HTML_Report_Image_Alignment."MIDDLE", "MS Office parameters"=T11 {"position (Excel)"={"row"=0, "column"=0}, "name (Excel)"="", "bookmark (Word)"="image"}, "path or URL of image"=w595) -> ("report out"=w591:refnum<class "NI_report.lvclass">, "error out"=w594:errorcluster)  [unwired: 8 in, 2 out]
                n347 = call <vilib>:"Word Easy Text.vi"("report in"=w591, "text"="检测结果：", "alignment (left)"=enum16{"Left", "Centered", "Right", "Justify"}."Left", "font"=T13 {"font name"="", "font size"=0.0, "bold"=0, "italic"=0, "underline"=0, "strike through"=0, "font color"=16777216}, "error in (no error)"=w592) -> ("report out"=w617:refnum<class "NI_report.lvclass">, "error out"=w618:errorcluster)  [unwired: 8 in, 1 out]
                n348 = case shown="错误" w594 {
                  frame No Error {
                  }
                  frame Error {
                    n349 = One Button Dialog(message="图片导入word\n发生错误！" ("消息")) -> ()  [unwired: 1 in, 1 out]
                  }
                }
                n350 = call-poly <vilib>:"Word Easy Table.vi"("report in"=w617, "column headers"=string[] ["框号", "X/mm", "Y/mm", "长/mm", "宽/mm", "面积/mm2", "Z值/mm", "部位", "类型", "合格性"], "data"=w608, "error in (no error)"=w618) -> ("report out"=w615:refnum<class "NI_report.lvclass">, "error out"=w614:errorcluster)  [unwired: 9 in, 1 out]
              }
              frame #4 {
                n351 = local read "穿透图原始路径"() -> (w627:path)
                n352 = local read "报告模式"() -> (w625:string)
                n353 = Path To String(path=w627) -> (string=w631:string)
                n354 = String Length(string=w631) -> (length=w632:i32)
                n355 = Subtract(x=w632, y=4) -> (x-y=w633:i32)
                n356 = Concatenate Strings("_" ("字符串"), w625, "_.docx" ("字符串")) -> (w623:string)
                n357 = Replace Substring(3:w633, 4:w623, 5:w631) -> (1:w630:string)  [unwired: 1 in, 1 out]
                n358 = String To Path(string=w630) -> (path=w628:path)
                "添加的路径" <- w628
                n359 = call-dynamic "Save Report to File.vi"("report in"=w635, "report file path"=w628, "prompt to replace? (F)"=TRUE, "error in (no error)"=w634) -> ("report out"=w639:refnum<class "NI_report.lvclass">, "error out"=w638:errorcluster)  [unwired: 10 in]
                n360 = call <vilib>:"Word Bring to Front.vi"("report in"=w639, "window state (maximized)"=enum16{"maximized", "minimized", "normal"}."normal", "error in (no error)"=w638) -> ()  [unwired: 11 in, 2 out]
              }
              frame #5 {
                n361 = local write "全部检测结果合并"(string[][] [] ("弥散类检测结果合并")) -> ()
                n362 = One Button Dialog(message="完成评定并退出程序！\n请查看word报告" ("消息")) -> ()  [unwired: 1 in, 1 out]
              }
            }
          }
        }
      }
      event "stop": Value Change {
        # "退出软件"
        n363 = event-data() -> ("NewVal"=w645:bool)  [unwired: 1 in, 4 out]
        n364 = Two Button Dialog(message="是否关闭本软件？" ("消息")) -> (T button?=w646:bool)  [unwired: 2 in]
        n365 = And(x=w645, y=w646) -> (x .and. y?=w644:bool)
        n366 = case shown="真" w644 {
          frame False {
          }
          frame True {
            w647 = TRUE ("All Images? (No)")
            n367 = local read "穿透图"() -> (w649:T1)
            n368 = local read "反射图"() -> (w648:T1)
            n369 = call "IMAQ Dispose"("All Images? (No)"=w647, "Image"=w649) -> ()  [unwired: 4 in, 1 out]
            n370 = call "IMAQ Dispose"("All Images? (No)"=w647, "Image"=w648) -> ()  [unwired: 4 in, 1 out]
            n371 = disable-structure shown="RUN_TIME_ENGINE==True" {
              frame condition #0 {
                n372 = Quit LabVIEW() -> ()  [unwired: 1 in]
              }
              frame condition #1 (active) {
                n373 = Stop() -> ()  [unwired: 1 in]
              }
            }
          }
        }
      }
    }
  }
  n374 = disable-structure shown="禁用" {
    frame Disabled {
      n375 = while {
        stop <- FALSE stop-if-true
        n376 = local read "查看评定结果"() -> (w652:bool)
        n377 = local read "删除标注"() -> (w653:bool)
        n378 = Or(x=w653, y=w652) -> (x .or. y?=w654:bool)
        n379 = local write "开始标注"(w654) -> ()
        n380 = Wait Until Next ms Multiple(millisecond multiple=u32 50 ("毫秒倍数")) -> ()  [unwired: 1 out]
      }
    }
    frame Enabled {
    }
  }
  n381 = disable-structure shown="禁用" {
    frame Disabled {
    }
    frame Enabled {
    }
  }
  "临界面积百分比值" <- w10
  "分层类缺陷灰度阈值" <- w11
  "弥散类缺陷灰度阈值" <- w1
